vi "Utest3.vi"() -> ()   [LabVIEW 2010]
panel:
  in  "Case Constant\n(See Context Help) 2":bool
  in  "Case Constant\n(See Context Help)":bool
  out "ModuleInfo":T1 {"DacScaleCoef" format="%#_2g"; "DacOffsetCoef" format="%#_2g"}
  out "InterfaceInfo":T2 {"ModuleHandle" format="%x"; "WriteBuffersParsArray"."WriteEvent" format="%x"; "WriteBuffersParsArray"."WriteOv" format="%x"; "ReadBuffersParsArray"."ReadEvent" format="%x"; "ReadBuffersParsArray"."ReadOv" format="%x"; "InterfaceType" items=["Unknown Module", "USB2185 Module", "USB3000 Module"]; "InterfaceInstance" format="%x"; "DllVersion" format="%x"}
  out "ViStatusOut":T3
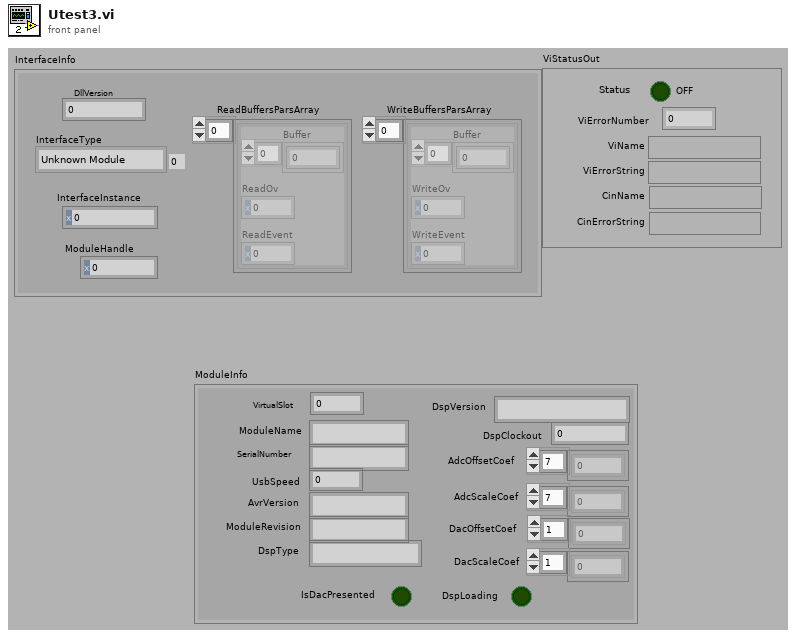
[diagram p1: front panel]
types:
  T1 = cluster{"VirtualSlot":u16, "ModuleName":string, "SerialNumber":string, "UsbSpeed":u8, "AvrVersion":string, "ModuleRevision":string, "DspType":string, "IsDacPresented":bool, "DspLoading":bool, "DspVersion":string, "DspClockout":u32, "AdcOffsetCoef":sgl[], "AdcScaleCoef":sgl[], "DacOffsetCoef":sgl[], "DacScaleCoef":sgl[]}
  T2 = cluster{"DllVersion":u32, "InterfaceType":u32, "InterfaceInstance":u32, "ModuleHandle":u32, "ReadBuffersParsArray":cluster{"Buffer":i16[], "ReadOv":u32, "ReadEvent":u32}[], "WriteBuffersParsArray":cluster{"Buffer":i16[], "WriteOv":u32, "WriteEvent":u32}[]}
  T3 = cluster{"Status":bool, "ViErrorNumber":u32, "ViName":string, "ViErrorString":string, "CinName":string, "CinErrorString":string}
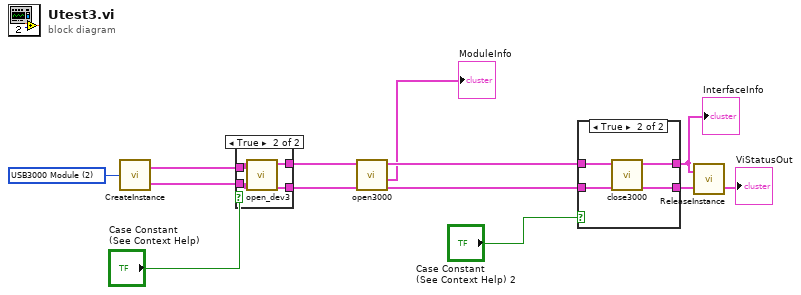
[diagram p0: block diagram]
diagram:
  w13 = u32 2 items=["Unknown Module", "USB2185 Module", "USB3000 Module"] ("InterfaceType")
  n1 = call "CreateInstance.vi"("InterfaceType"=w13) -> ("InterfaceInfo"=w11:T2, "ViStatus"=w10:T3)
  n2 = case shown="True" "Case Constant\n(See Context Help)" {
    tunnel: w11 -> [w15 w19]
    tunnel: w10 -> [w14 w18]
    tunnel: [w15 w17] -> w5
    tunnel: [w14 w16] -> w4
    frame False {
    }
    frame True {
      n3 = call "open_dev3.vi"("ViStatus"=w18, "InterfaceInfo 2"=w19) -> ("ViStatus 2"=w16:T3, "InterfaceInfo"=w17:T2)  [unwired: 2 in, 2 out]
    }
  }
  n4 = call "open3000.vi"("ViInfo"=w4, "InterfaceInfo"=w5) -> ("ViInfoOut"=w2:T3, "ModuleInfo"=→"ModuleInfo":T1, "InterfaceInfoOut"=w3:T2)  [unwired: 3 in]
  n5 = case shown="True" "Case Constant\n(See Context Help) 2" {
    tunnel: [w20 w25] -> w9
    tunnel: [w21 w24] -> w8
    tunnel: w3 -> [w21 w23]
    tunnel: w2 -> [w20 w22]
    frame False {
    }
    frame True {
      n6 = call "close3000.vi"("ViStatus"=w22, "InterfaceInfo"=w23) -> ("ViStatusOut"=w25:T3, "InterfaceInfoOut"=w24:T2)  [unwired: 4 in]
    }
  }
  "InterfaceInfo" <- w8
  n7 = call "ReleaseInstance.vi"("ViStatusIn"=w9, "InterfaceInfoIn"=w8) -> ("ViStatusOut"=→"ViStatusOut":T3)  [unwired: 1 out]
